vi "Move Digital Pattern to RIO.vi"(6 "New RIO":string, 8 "error in (no error)":errorcluster, 9 "Name":string, 10 "Old RIO":string, 11 "Item Ref in":T1 format="%.0x") -> (0 "error out":errorcluster, 2 "Digital Pattern Ref out":T1 format="%.0x", 3 "Item Ref out":T1 format="%.0x")   [LabVIEW 2020, in "Engine Simulation Toolkit System Explorer.lvlib"]
uses:
  Engine Simulation Toolkit System Explorer.lvlib
  <vilib>/NI VeriStand/Custom Device API/Custom Device Item Ref.ctl
  <vilib>/NI VeriStand/Custom Device API/Custom Device API.lvlib
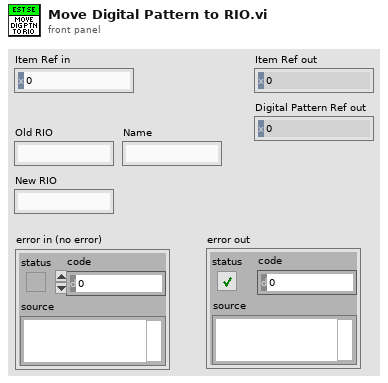
[diagram p1: front panel]
types:
  T1 = typedef "Custom Device API.lvlib/Custom Device Item Ref.ctl" = u64
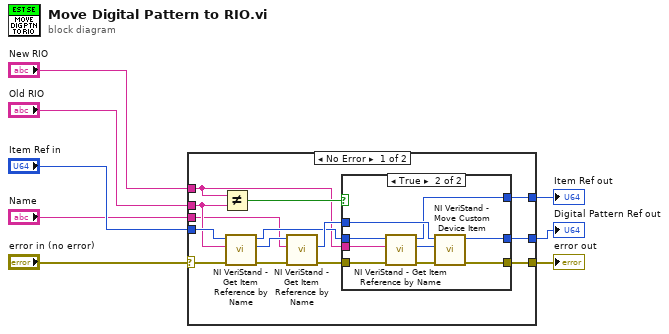
[diagram p0: block diagram]
diagram:
  n1 = case shown="No Error" "error in (no error)" {
    selector: "error in (no error)" -> [w16 w36]
    tunnel: [w15 w36] -> w7
    tunnel: "Item Ref in" -> [w14 w35]
    tunnel: [w13 w35] -> w5
    tunnel: "New RIO" -> [w12 _]
    tunnel: "Old RIO" -> [w11 _]
    tunnel: "Name" -> [w10 _]
    tunnel: [w9 _] -> w1
    frame No Error {
      n2 = Not Equal?(x=w12, y=w11) -> (x != y?=w17:bool)
      n3 = call <vilib>:"NI VeriStand - Get Item Reference by Name.vi"("error in (no error)"=w16, "Item Name"=w11, "Parent Ref in"=w14) -> ("error out"=w21:errorcluster, "Item Ref"=w22:T1, "Parent Ref out"=w18:T1)  [unwired: 5 in, 1 out]
      n4 = call <vilib>:"NI VeriStand - Get Item Reference by Name.vi"("error in (no error)"=w21, "Item Name"=w10, "Parent Ref in"=w22) -> ("error out"=w20:errorcluster, "Item Ref"=w19:T1)  [unwired: 5 in, 2 out]
      n5 = case shown="True" w17 {
        tunnel: [w25 w34] -> w15
        tunnel: w12 -> [_ w33]
        tunnel: w20 -> [w25 w32]
        tunnel: w19 -> [w24 w31]
        tunnel: w18 -> [w23 w28]
        tunnel: [w23 w27] -> w13
        tunnel: [w24 w26] -> w9
        frame False {
          # "Already parented\ncorrectly"
        }
        frame True {
          n6 = call <vilib>:"NI VeriStand - Get Item Reference by Name.vi"("error in (no error)"=w32, "Item Name"=w33, "Parent Ref in"=w28) -> ("error out"=w29:errorcluster, "Item Ref"=w30:T1, "Parent Ref out"=w27:T1)  [unwired: 5 in, 1 out]
          n7 = call <vilib>:"NI VeriStand - Move Custom Device Item.vi"("error in (no error)"=w29, "New Parent Ref in"=w30, "Item Ref in"=w31) -> ("error out"=w34:errorcluster, "Item Ref out"=w26:T1)  [unwired: 6 in, 1 out]
        }
      }
    }
    frame Error {
    }
  }
  "error out" <- w7
  "Item Ref out" <- w5
  "Digital Pattern Ref out" <- w1
